vi "Main.vi"() -> ()   [LabVIEW 2024]
doc: "This VI demonstrates how LabVIEW can use the drivers provided by MotioninJoy software to make full use of a Dualshock 3 Playstation 3 controller. It uses a type definition which allows a user to see direct button mapping."
uses:
  Controls/PS3 Controls.ctl
  <vilib>/Utility/inputDevices.llb/closeJoystick.vi
panel:
  in  "stop":bool
  out "PS3 Controls":T1 {"Left Analogue Stick X" scale=-32768.0..32768.0; "Left Analogue Stick Y" scale=32768.0..-32768.0; "Right Analogue Stick X" scale=-32768.0..32768.0; "Right Analogue Stick Y" scale=32768.0..-32768.0; "X Rotation" scale=-32768.0..32768.0; "Y Rotation" scale=-32768.0..32768.0; "L2 Pressure" scale=0.0..32768.0; "Numeric" format="%d°"}
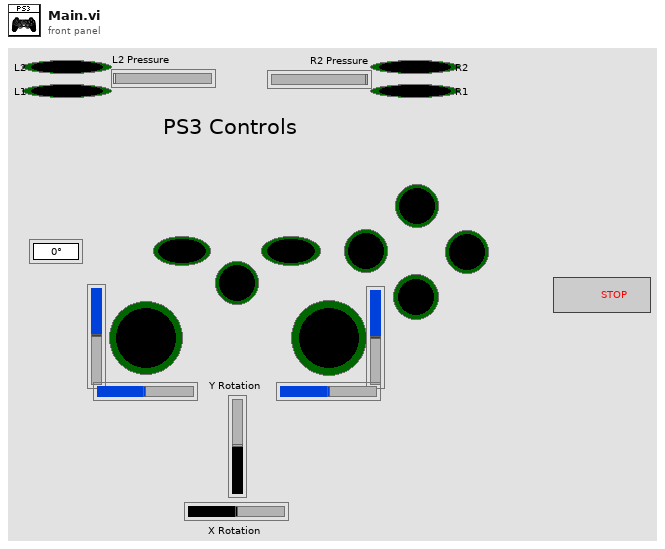
[diagram p1: front panel]
types:
  T1 = typedef "PS3 Controls.ctl" = cluster{"Left Analogue Stick X":i32, "Left Analogue Stick Y":i32, "Right Analogue Stick X":i32, "Right Analogue Stick Y":i32, "Y Rotation":i32, "X Rotation":i32, "L2 Pressure":i32, "R2 Pressure":i32, "Triangle":bool, "Circle":bool, "X":bool, "Square":bool, "L1":bool, "R1":bool, "L2":bool, "R2":bool, "L3":bool, "R3":bool, "Select":bool, "Start":bool, "PS Button":bool, "Numeric":i32}
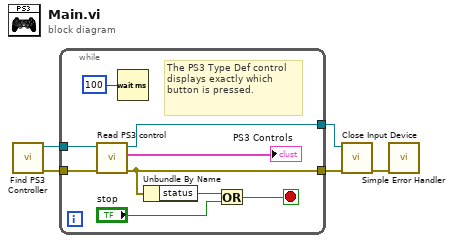
[diagram p0: block diagram]
diagram:
  n1 = call "Find PS3 Controller.vi"() -> ("error out"=w5:errorcluster, "Controller Reference Out"=w4:refnum<k1>)  [unwired: 9 in, 1 out]
  n2 = while {
    tunnel: w5 -> [w11]
    tunnel: w4 -> [w10]
    tunnel: [w9] -> w2
    tunnel: [w7] -> w1
    stop <- w13 stop-if-true
    # "The PS3 Type Def control displays exactly which button is pressed."
    n3 = call "Read PS3 control.vi"("error in (no error)"=w11, "Controller Reference In"=w10) -> ("error out"=w7:errorcluster, "PS3 Controls"=→"PS3 Controls":T1, "Controller Reference Out"=w9:refnum<k1>)  [unwired: 7 in]
    n4 = Wait (ms)(milliseconds to wait=u32 100) -> ()  [unwired: 1 out]
    n5 = Unbundle By Name(w7) -> ("status"=w6:bool)
    n6 = Or(x=w6, y="stop") -> (x .or. y?=w13:bool)
  }
  n7 = call-poly <vilib>:"Close Input Device.vi"("error in (no error)"=w1, "device ID"=w2) -> ("error out"=w3:errorcluster)  [unwired: 8 in]
  n8 = call <vilib>:"Simple Error Handler.vi"("error in (no error)"=w3) -> ()  [unwired: 4 in, 5 out]
